vi "configuration_rm_depth_ahat.vi"() -> (3 "configuration_rm_depth_ahat":T1)   [LabVIEW 2023]
panel:
  in  "configuration_rm_depth_ahat":T1={"chunk"=4096, "mode"=1, "divisor"=1, "profile_z"=0, "profile_ab"=3, "level"=255, "_reserved_0"=0, "_reserved_1"=0, "_reserved_2"=0, "bitrate"=0, "_reserved_3"=0, "options_size"=-1, "options_data"=0, "_reserved_4"=0}
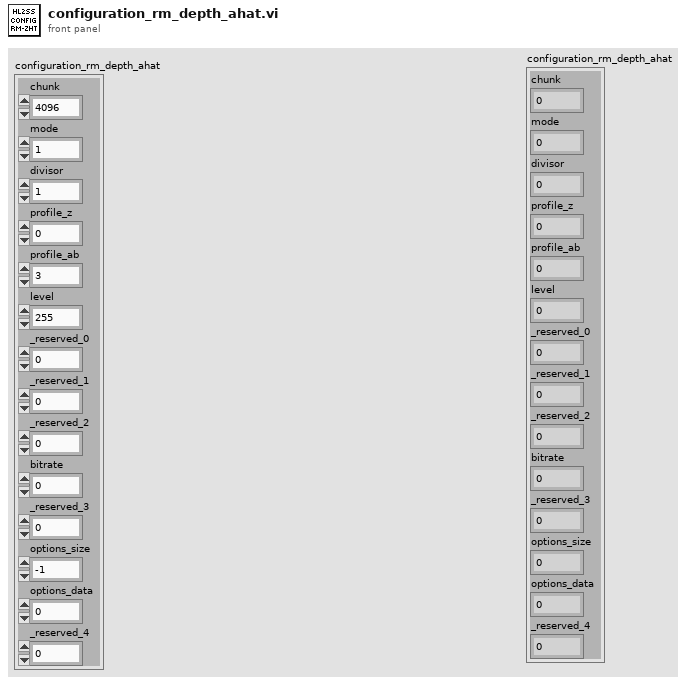
[diagram p1: front panel]
types:
  T1 = cluster{"chunk":u64, "mode":u8, "divisor":u8, "profile_z":u8, "profile_ab":u8, "level":u8, "_reserved_0":u8, "_reserved_1":u8, "_reserved_2":u8, "bitrate":u32, "_reserved_3":u32, "options_size":i64, "options_data":u64, "_reserved_4":u64}
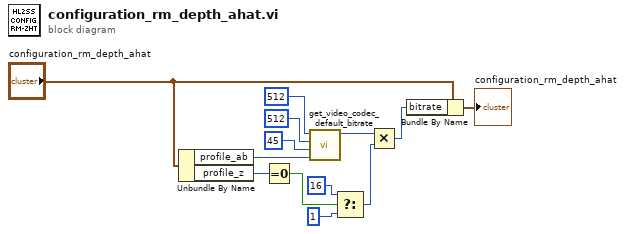
[diagram p0: block diagram]
diagram:
  n1 = Unbundle By Name("configuration_rm_depth_ahat") -> ("profile_ab"=w10:u8, "profile_z"=w3:u8)
  n2 = Equal To 0?(x=w3) -> (x = 0?=w2:bool)
  n3 = call "get_video_codec_default_bitrate.vi"("profile"=w10, "framerate"=u8 45, "height"=u16 512, "width"=u16 512) -> ("bitrate"=w9:u32)  [unwired: 7 in]
  n4 = Select(t=u32 16, s=w2, f=u32 1) -> (s? t:f=w6:u32)
  n5 = Multiply(x=w9, y=w6) -> (x*y=w4:u32)
  n6 = Bundle By Name(cluster="configuration_rm_depth_ahat", "bitrate"=w4) -> (→"configuration_rm_depth_ahat":T1)
